vi "Find One Cycle R1.vi"(11 "data in":i32[][](array[numeric])) -> (1 "n crossings":i32, 3 "data out":i32[][](array[numeric]))   [LabVIEW 2018]
uses:
  <vilib>/ptbypt/NI_PtbyPt.lvlib
panel:
  in  "Trigger":enum16{"either", "minus-plus", "plus-minus"}(ring)
  out "Loop Iterations":i32
  out "crossing indices":i32[](array[numeric])
  out "Plotting Data":i32[](graph) caption="Waveform Chart - dark"
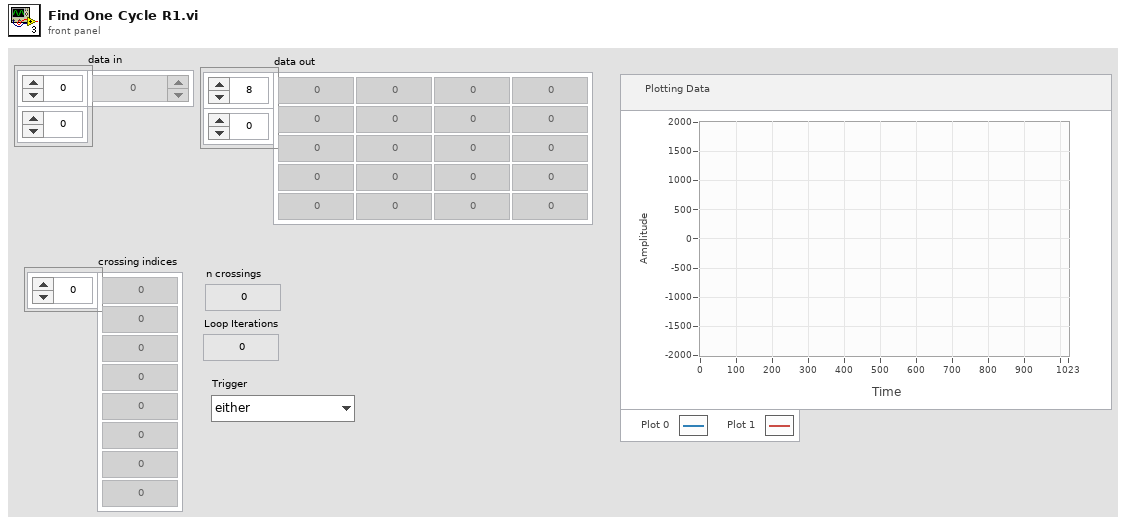
[diagram p1: front panel]
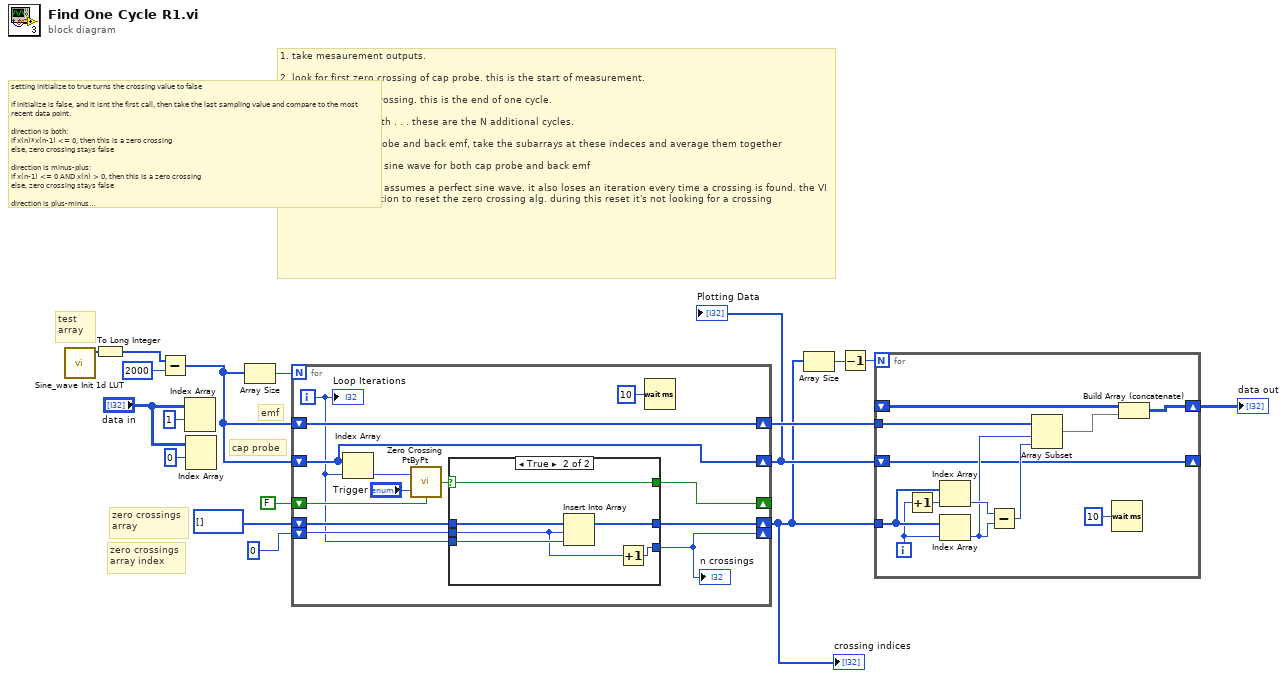
[diagram p0: block diagram]
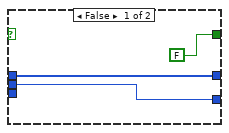
[diagram p2: hidden frame]
diagram:
  # "setting initialize to true turns the crossing value to false\n\nif initialize is false, and it isnt the first call, then take the last sampling value and compare to the most recent data point.\n\ndirection is both:\nif x(n)*x(n-1) <= 0, then this is a zero crossing\nelse, zero crossing stays false\n\ndirection is minus-plus:\nif x(n-1) <= 0 AND x(n) > 0, then this is a zero crossing\nelse, zero crossing stays false\n\ndirection is plus-minus\nif x(n-1) > 0 AND x(n) <= 0, then this is a zero crossing\nelse, zero crossing stays false"
  # "test\narray"
  # "cap probe"
  # "emf"
  # "zero crossings\narray index"
  # "zero crossings\narray"
  # "1. take mesaurement outputs.\n\n2. look for first zero crossing of cap probe. this is the start of measurement.\n\n3. look for 3rd zero crossing. this is the end of one cycle.\n\n4. look for 5th, 7th, 9th . . . these are the N additional cycles.\n\n5. for both the cap probe and back emf, take the subarrays at these indeces and average them together\n\n6. output a one-cycle sine wave for both cap probe and back emf\n\nthis code, as written, assumes a perfect sine wave. it also loses an iteration every time a crossing is found. the VI needs one loop iteration to reset the zero crossing alg. during this reset it's not looking for a crossing"
  n1 = call "Sine_wave Init 1d LUT.vi"() -> ("Init Data Out"=w8:u16[])  [unwired: 11 in]
  n2 = To Long Integer(number=w8) -> (32bit integer=w10:i32[])
  n3 = Subtract(x=w10, y=2000 ("index (row)")) -> (x-y=w7:i32[])
  n4 = Index Array(array="data in", index (row)=1) -> ()  [unwired: 1 in, 1 out]
  n5 = Index Array(array="data in", index (row)=0) -> ()  [unwired: 1 in, 1 out]
  n6 = Array Size(array=w7) -> (size(s)=w14:i32)
  n7 = for {
    N: w14 -> [_]
    shift-right: [w25] -> w5
    shift-left: w7 -> [w25]
    shift-right: [w27] -> w6
    shift-left: w7 -> [w27]
    shift-right: [w30] -> w2
    shift-left: i32[] [] ("subarray") -> [w28]
    shift-right: [w21] -> _
    shift-left: 0 ("n cycles") -> [w29]
    shift-right: [w24] -> _
    shift-left: FALSE -> [w23]
    i -> [w19]
    n8 = Index Array(array=w25, index=w19) -> (element=w26:i32)
    n9 = call <vilib>:"Zero Crossing PtByPt.vi"("initialize"=w23, "direction"="Trigger", "input data point"=w26) -> ("crossing"=w20:bool)
    n10 = case shown="True" w20 {
      selector: w20 -> [_ w36]
      tunnel: [w33 w39] -> w21
      tunnel: [w32 w37] -> w30
      tunnel: w29 -> [w33 w34]
      tunnel: w28 -> [w32 w38]
      tunnel: [FALSE w36] -> w24
      tunnel: w19 -> [_ w35]
      frame False {
      }
      frame True {
        n11 = Insert Into Array(array=w38, index=w34, new element=w35) -> (w37:i32[])
        n12 = Increment(x=w34) -> (x+1=w39:i32)
      }
    }
    "n crossings" <- w21
    n13 = Wait (ms)(milliseconds to wait=u32 10) -> ()  [unwired: 1 out]
    "Loop Iterations" <- w19
  }
  "Plotting Data" <- w5
  "crossing indices" <- w2
  n14 = Array Size(array=w2) -> (size(s)=w4:i32)
  n15 = Decrement(x=w4) -> (x-1=w3:i32)
  n16 = for {
    N: w3 -> [_]
    shift-right: [w42] -> _
    shift-left: w5 -> [w42]
    tunnel: w6 -> [w51]
    shift-right: [w40] -> w1
    shift-left: _ -> [w43]
    tunnel: w2 -> [w50]
    i -> [w49]
    n17 = Increment(x=w49) -> (x+1=w48:i32)
    n18 = Index Array(array=w50, index=w48) -> (element=w46:i32)
    n19 = Index Array(array=w50, index=w49) -> (element=w45:i32)
    n20 = Subtract(x=w46, y=w45) -> (x-y=w47:i32)
    n21 = Array Subset(array=w51, index=w45, length=w47) -> (w44:i32[])
    n22 = Wait (ms)(milliseconds to wait=u32 10) -> ()  [unwired: 1 out]
    n23 = Build Array (concatenate)(w43, w44) -> (w40:i32[][])
  }
  "data out" <- w1
